vi "Float32Array Create (Dimensions).vi"(8 "error in (no error)":errorcluster, 10 "Array dimensions":i32[](array[numeric]), 11 "SGL array in":sgl[](array[numeric])) -> (0 "error out":errorcluster, 3 "Float32Array DVR out":refnum<data-value>)   [LabVIEW 2015, in "MDSplus.lvlib"]
uses:
  <vilib>/MDSplus/Library/MDSplus.lvlib
  <vilib>/MDSplus/Classes/Data_Class/Array_Class/Float32Array_Class/Float32Array.lvclass
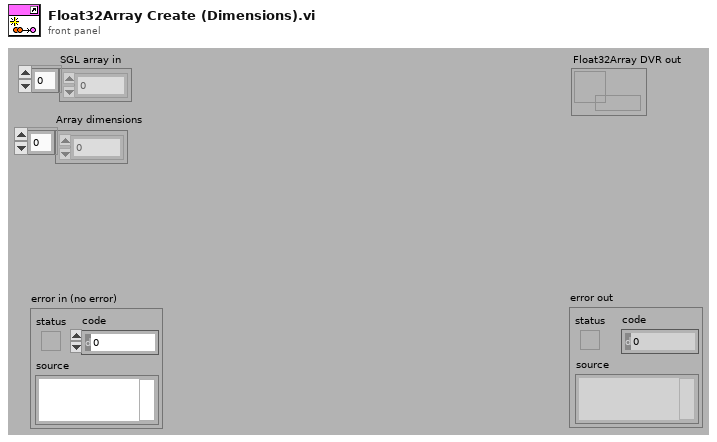
[diagram p1: front panel]
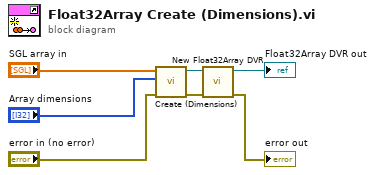
[diagram p0: block diagram]
diagram:
  n1 = call <vilib>:"Create (Dimensions).vi"("error in (no error)"="error in (no error)", "Dimensions"="Array dimensions", "SGL array in"="SGL array in") -> ("error out"=w4:errorcluster, "Float32Array out"=w5:refnum<class "Float32Array.lvclass">)  [unwired: 7 in]
  n2 = call <vilib>:"New Float32Array DVR.vi"("error in (no error)"=w4, "Float32Array in"=w5) -> ("error out"=→"error out":errorcluster, "Float32Array DVR out"=→"Float32Array DVR out":refnum<data-value>)  [unwired: 8 in]
